vi "BERT Measurement Result.vi"(0 "VISA Resource Name":refnum<visa-resource-name>, 5 "Var (0:Intermed Bit Error Cnt)":T1(ring), 11 "error in (no error)":errorcluster {"code" format="%.0x"}) -> (4 "VISA Resource Name Out":refnum<visa-resource-name>, 6 "Result":string, 15 "error out":errorcluster {"code" format="%.0x"})   [LabVIEW 2012, in "Agilent ESG Series.lvlib"]
doc: "This VI is used to read the measurement result value."
uses:
  <instrlib>/Agilent ESG Series/Agilent ESG Series.lvlib
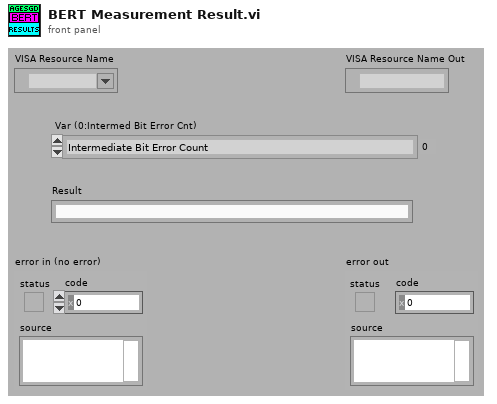
[diagram p1: front panel]
types:
  T1 = enum16{"Intermediate Bit Error Count", "Intermediate Bit Error Rate", "Intermediate Bit Count", "Pass/Fail result", "Total Bit Error Count at the one measurement cycle end", "Total Bit Error Rate at one measurement cycle end", "Total Bit Count at the one measurement cycle end"}
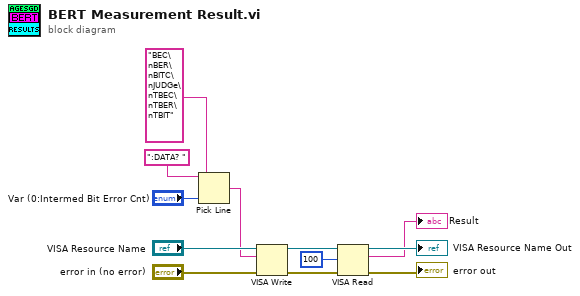
[diagram p0: block diagram]
diagram:
  n1 = Pick Line(string ("")=":DATA? ", multi-line string="BEC\nBER\nBITC\nJUDGe\nTBEC\nTBER\nTBIT", line index="Var (0:Intermed Bit Error Cnt)") -> (output string=w1:string)
  n2 = VISA Write(VISA resource name="VISA Resource Name", write buffer=w1, error in (no error)="error in (no error)") -> (VISA resource name out=w7:refnum<visa-resource-name>, error out=w6:errorcluster)  [unwired: 1 out]
  n3 = VISA Read(VISA resource name=w7, byte count=u32 100 ("byte count (0)"), error in (no error)=w6) -> (VISA resource name out=→"VISA Resource Name Out":refnum<visa-resource-name>, read buffer=→"Result":string, error out=→"error out":errorcluster)  [unwired: 1 out]
